vi "loadSubVIfromRef.vi"(8 "error in (no error)":errorcluster, 9 "DataNode*":refnum<data-value>, 10 "RootNode*":refnum<data-value>, 11 "xceSubPanel in":refnum<class "xceSubPanel.lvclass">) -> (0 "error out":errorcluster, 3 "xceSubPanel out":refnum<class "xceSubPanel.lvclass">)   [LabVIEW 2013, in "xceSubPanel.lvclass"]
doc: "Loads a User Interface VI from a particular node in the tree data structure."
uses:
  xceSubPanel.lvclass
  xceRootNode/xceRootNode.lvclass
  xceDataNode/xceDataNode.lvclass
  xceSubPanel.lvclass/xceSubPanel.ctl
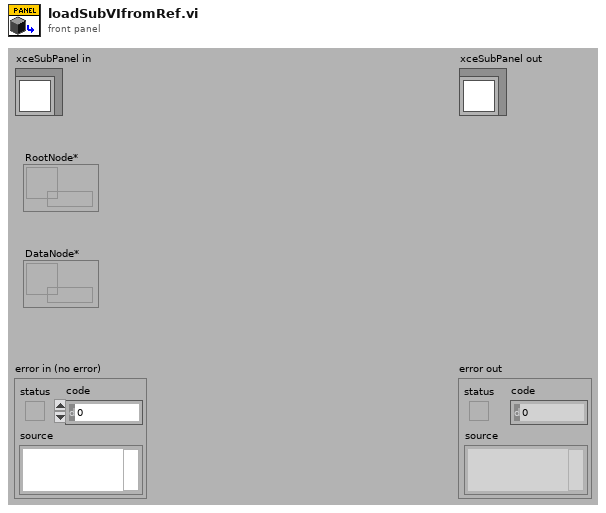
[diagram p1: front panel]
types:
  T1 = typedef "AMC.lvlib/Message Queue.ctl" = refnum<queue>
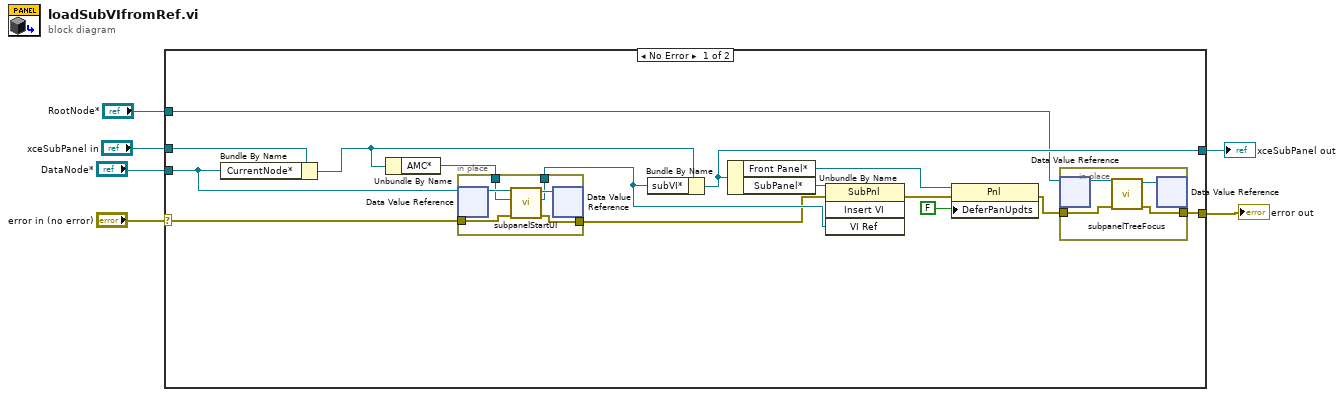
[diagram p0: block diagram]
diagram:
  n1 = case shown="No Error" "error in (no error)" {
    selector: "error in (no error)" -> [w11 w33]
    tunnel: [w8 w33] -> w5
    tunnel: [w10 w32] -> w3
    tunnel: "xceSubPanel in" -> [w12 w32]
    tunnel: "DataNode*" -> [w7 _]
    tunnel: "RootNode*" -> [w9 _]
    frame No Error {
      n2 = Bundle By Name(cluster=w12, "CurrentNode*"=w7) -> (w17:refnum<class "xceSubPanel.lvclass">)
      n3 = Unbundle By Name(w17) -> ("AMC*"=w19:T1)
      n4 = in-place {
        in-place-border: w11 -> [w29]
        in-place-border: [w28] -> w16
        in-place-border: w19 -> [w27]
        in-place-border: [w26] -> w18
        n5 = in-place-dvr #1(w7) -> (w31:refnum<class "xceDataNode.lvclass">)  [unwired: 1 out]
        n6 = call "subpanelStartUI.vi"("error in (no error)"=w29, "AMC*"=w27, "xceDataNode in"=w31) -> ("error out"=w28:errorcluster, "UI VI*"=w26:refnum<vi>, "xceDataNode out"=w30:refnum<class "xceDataNode.lvclass">)  [unwired: 6 in]
        n7 = in-place-dvr #1(w30) -> ()  [unwired: 2 out]
      }
      n8 = Bundle By Name(cluster=w17, "subVI*"=w18) -> (w10:refnum<class "xceSubPanel.lvclass">)
      n9 = Unbundle By Name(w10) -> ("Front Panel*"=w15:refnum<vi>, "SubPanel*"=w21:refnum<vi>)
      n10 = invoke class="SubPnl" method="Insert VI"(reference=w21, error in=w16, "VI Ref"=w18) -> (error out=w14:errorcluster)  [unwired: 1 in, 3 out]
      n11 = property class="Pnl"(reference=w15, error in=w14, "DeferPanUpdts"=FALSE ("Defer Panel Updates")) -> (error out=w13:errorcluster)  [unwired: 1 out]
      n12 = in-place {
        in-place-border: w13 -> [w23]
        in-place-border: [w22] -> w8
        n13 = in-place-dvr #2(w9) -> (w25:refnum<class "xceRootNode.lvclass">)  [unwired: 1 out]
        n14 = call "subpanelTreeFocus.vi"("error in (no error)"=w23, "xceRootNode in"=w25) -> ("error out"=w22:errorcluster, "xceRootNode out"=w24:refnum<class "xceRootNode.lvclass">)  [unwired: 8 in]
        n15 = in-place-dvr #2(w24) -> ()  [unwired: 2 out]
      }
    }
    frame Error {
    }
  }
  "error out" <- w5
  "xceSubPanel out" <- w3
